vi "cwlaserShutterOpenOneCloseOthers.vi"(1 "wavelength":dbl) -> ()   [LabVIEW 2017]
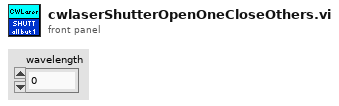
[diagram p1: front panel]
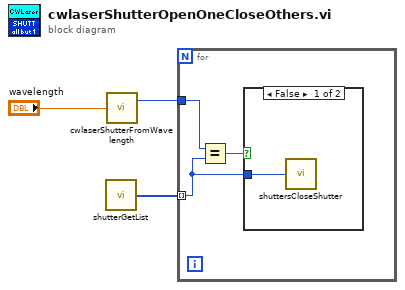
[diagram p0: block diagram]
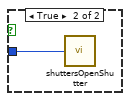
[diagram p2: hidden frame]
diagram:
  n1 = call "shutterGetList.vi"() -> ("list of shutters"=w2:i32[])  [unwired: 1 in]
  n2 = call "cwlaserShutterFromWavelength.vi"("wavelength (nm)"="wavelength") -> ("shutter"=w1:i32)  [unwired: 1 out]
  n3 = for {
    tunnel: w2 -> [w4] mode=indexing
    tunnel: w1 -> [w6]
    n4 = Equal?(x=w6, y=w4) -> (x = y?=w5:bool)
    n5 = case shown="False" w5 {
      tunnel: w4 -> [w7 w8]
      frame False {
        n6 = call "shuttersCloseShutter.vi"("shutter"=w7) -> ()  [unwired: 1 in]
      }
      frame True {
        n7 = call "shuttersOpenShutter.vi"("shutter"=w8) -> ()  [unwired: 1 in]
      }
    }
  }
